vi "Configure Library on Disk for Build.vi"(9 "enable debugging? (F)":bool, 10 "save VIs? (T)":bool=TRUE, 11 "library path":path) -> (0 "error out":errorcluster)   [LabVIEW 2019, in "Build Automation.lvlib"]
uses:
  Build Automation.lvlib
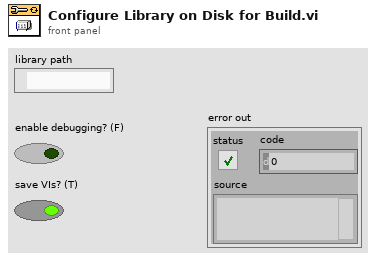
[diagram p1: front panel]
types:
  T1 = enum16{"Share clones between instances", "Preallocate clone for each instance"}
  T2 = cluster{"Status Message":refnum<data-value>, "Progress":refnum<data-value>, "Stop":refnum<data-value>}
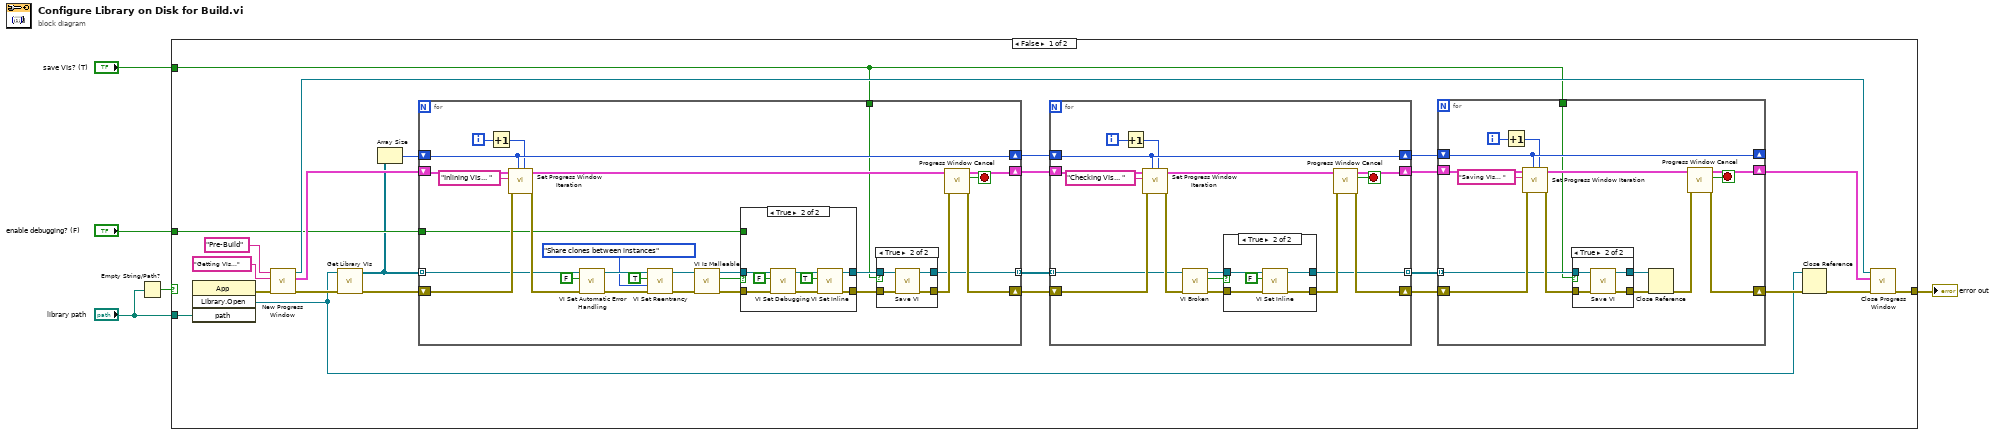
[diagram p0: block diagram]
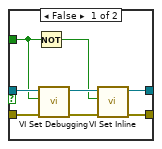
[diagram p3: hidden frame]
diagram:
  n1 = Empty String/Path?(string/path="library path") -> (empty?=w3:bool)
  n2 = case shown="False" w3 {
    tunnel: [w26 _] -> w5
    tunnel: "enable debugging? (F)" -> [w25 _]
    tunnel: "save VIs? (T)" -> [w7 _]
    tunnel: "library path" -> [w8 _]
    frame False {
      n3 = invoke class="App" method="Library.Open"("path"=w8) -> (error out=w9:errorcluster, "Open Library"=w10:refnum<vi>)  [unwired: 3 in, 2 out]
      n4 = call "New Progress Window.vi"("error in (no error)"=w9, "Initial Message"="Getting VIs...", "Window Title"="Pre-Build" ("WindowTitle")) -> ("error out"=w28:errorcluster, "DVRs"=w27:T2, "VI refnum"=w29:refnum<vi>)  [unwired: 6 in]
      n5 = call "Get Library VIs.vi"("error in (no error)"=w28, "library ref"=w10) -> ("error out"=w30:errorcluster, "vi refs"=w23:refnum<vi>[])  [unwired: 8 in]
      n6 = Array Size(array=w23) -> (size(s)=w24:i32)
      n7 = for {
        tunnel: w23 -> [w42] mode=indexing
        shift-right: [w56] -> w21
        shift-left: w27 -> [w47]
        shift-right: [w43] -> w19
        shift-left: w30 -> [w45]
        tunnel: w25 -> [w41]
        tunnel: [w34] -> w20 mode=indexing
        shift-right: [w40] -> w22
        shift-left: w24 -> [w40]
        tunnel: w7 -> [w33]
        i -> [w58]
        stop <- w57 stop-if-true
        n8 = Increment(x=w58) -> (x+1=w39:i32)
        n9 = call "Set Progress Window Iteration.vi"("current iteration"=w39, "total iterations"=w40, "error in (no error)"=w45, "Status Message"="Inlining VIs... ", "DVRs in"=w47) -> ("error out"=w44:errorcluster, "DVRs out"=w46:T2)  [unwired: 5 in]
        n10 = call "VI Set Automatic Error Handling.vi"("error in (no error)"=w44, "Automatic Error Handling"=FALSE, "vi ref in"=w42) -> ("error out"=w53:errorcluster, "vi ref out"=w54:refnum<vi>)  [unwired: 7 in]
        n11 = call "VI Set Reentrancy.vi"("error in (no error)"=w53, "Reentrancy Type (shared clone)"=T1."Share clones between instances" ("Reentrancy Type"), "Is Reentrant"=TRUE, "vi ref in"=w54) -> ("error out"=w51:errorcluster, "vi ref out"=w52:refnum<vi>)  [unwired: 6 in]
        n12 = call "VI Is Malleable.vi"("error in (no error)"=w51, "vi ref in"=w52) -> ("error out"=w50:errorcluster, "malleable VI?"=w48:bool, "vi ref out"=w49:refnum<vi>)  [unwired: 7 in]
        n13 = case shown="True" w48 {
          tunnel: [w70 w78] -> w36
          tunnel: [w69 w77] -> w37
          tunnel: w50 -> [w66 w75]
          tunnel: w49 -> [w67 w76]
          tunnel: w41 -> [w65 _]
          frame False {
            n14 = Not(x=w65) -> (.not. x?=w68:bool)
            n15 = call "VI Set Debugging.vi"("error in (no error)"=w66, "Allow Debugging"=w65, "vi ref in"=w67) -> ("error out"=w71:errorcluster, "vi ref out"=w72:refnum<vi>)  [unwired: 7 in]
            n16 = call "VI Set Inline.vi"("error in (no error)"=w71, "Inline VI"=w68, "vi ref in"=w72) -> ("error out"=w69:errorcluster, "vi ref out"=w70:refnum<vi>)  [unwired: 7 in]
          }
          frame True {
            n17 = call "VI Set Debugging.vi"("error in (no error)"=w75, "Allow Debugging"=FALSE, "vi ref in"=w76) -> ("error out"=w79:errorcluster, "vi ref out"=w80:refnum<vi>)  [unwired: 7 in]
            n18 = call "VI Set Inline.vi"("error in (no error)"=w79, "Inline VI"=TRUE, "vi ref in"=w80) -> ("error out"=w77:errorcluster, "vi ref out"=w78:refnum<vi>)  [unwired: 7 in]
          }
        }
        n19 = case shown="True" w33 {
          tunnel: w37 -> [w59 w64]
          tunnel: [w60 w63] -> w34
          tunnel: [w59 w62] -> w35
          tunnel: w36 -> [w60 w61]
          frame False {
          }
          frame True {
            n20 = call "Save VI.vi"("error in (no error)"=w64, "vi ref in"=w61) -> ("error out"=w62:errorcluster, "vi ref out"=w63:refnum<vi>)  [unwired: 8 in]
          }
        }
        n21 = call "Progress Window Cancel.vi"("error in (no error)"=w35, "DVRs in"=w46) -> ("error out"=w43:errorcluster, "cancelled"=w57:bool, "DVRs out"=w56:T2)  [unwired: 7 in]
      }
      n22 = for {
        tunnel: w20 -> [w86] mode=indexing
        shift-right: [w95] -> w18
        shift-left: w21 -> [w94]
        shift-right: [w91] -> w16
        shift-left: w19 -> [w92]
        shift-right: [w90] -> w17
        shift-left: w22 -> [w90]
        tunnel: [w81] -> w15 mode=indexing
        i -> [w97]
        stop <- w96 stop-if-true
        n23 = Increment(x=w97) -> (x+1=w89:i32)
        n24 = call "Set Progress Window Iteration.vi"("current iteration"=w89, "total iterations"=w90, "error in (no error)"=w92, "Status Message"="Checking VIs... ", "DVRs in"=w94) -> ("error out"=w87:errorcluster, "DVRs out"=w93:T2)  [unwired: 5 in]
        n25 = call "VI Broken.vi"("error in (no error)"=w87, "vi ref in"=w86) -> ("error out"=w84:errorcluster, "broken?"=w83:bool, "vi ref out"=w85:refnum<vi>)  [unwired: 7 in]
        n26 = case shown="True" w83 {
          tunnel: [w99 w104] -> w81
          tunnel: [w98 w103] -> w82
          tunnel: w84 -> [w98 w102]
          tunnel: w85 -> [w99 w100]
          frame False {
          }
          frame True {
            n27 = call "VI Set Inline.vi"("error in (no error)"=w102, "Inline VI"=FALSE, "vi ref in"=w100) -> ("error out"=w103:errorcluster, "vi ref out"=w104:refnum<vi>)  [unwired: 7 in]
          }
        }
        n28 = call "Progress Window Cancel.vi"("error in (no error)"=w82, "DVRs in"=w93) -> ("error out"=w91:errorcluster, "cancelled"=w96:bool, "DVRs out"=w95:T2)  [unwired: 7 in]
      }
      n29 = for {
        tunnel: w15 -> [w106] mode=indexing
        shift-right: [w118] -> w14
        shift-left: w18 -> [w117]
        shift-right: [w114] -> w12
        shift-left: w16 -> [w115]
        shift-right: [w113] -> _
        shift-left: w17 -> [w113]
        tunnel: w7 -> [w105]
        i -> [w120]
        stop <- w119 stop-if-true
        n30 = Increment(x=w120) -> (x+1=w112:i32)
        n31 = call "Set Progress Window Iteration.vi"("current iteration"=w112, "total iterations"=w113, "error in (no error)"=w115, "Status Message"="Saving VIs... ", "DVRs in"=w117) -> ("error out"=w107:errorcluster, "DVRs out"=w116:T2)  [unwired: 5 in]
        n32 = case shown="True" w105 {
          tunnel: w107 -> [w121 w126]
          tunnel: [w122 w125] -> w110
          tunnel: [w121 w124] -> w109
          tunnel: w106 -> [w122 w123]
          frame False {
          }
          frame True {
            n33 = call "Save VI.vi"("error in (no error)"=w126, "vi ref in"=w123) -> ("error out"=w124:errorcluster, "vi ref out"=w125:refnum<vi>)  [unwired: 8 in]
          }
        }
        n34 = Close Reference(reference=w110, error in (no error)=w109) -> (error out=w108:errorcluster)
        n35 = call "Progress Window Cancel.vi"("error in (no error)"=w108, "DVRs in"=w116) -> ("error out"=w114:errorcluster, "cancelled"=w119:bool, "DVRs out"=w118:T2)  [unwired: 7 in]
      }
      n36 = Close Reference(reference=w10, error in (no error)=w12) -> (error out=w11:errorcluster)
      n37 = call "Close Progress Window.vi"("error in (no error)"=w11, "DVRs in"=w14, "VI refnum"=w29) -> ("error out"=w26:errorcluster)  [unwired: 8 in]
    }
    frame True {
    }
  }
  "error out" <- w5
